vi "Plot area resize.vi"(8 "error in (no error)":errorcluster, 11 "Refs":T1) -> (0 "error out":errorcluster)   [LabVIEW 2021, in "RocketPlot.lvlib"]
uses:
  RocketPlot.lvlib
  TypeDefs/Plot UI references.ctl
  Classes/RocketPlotHandle/RocketPlotHandle.lvclass
  <userlib>/bjustice/TipStripOOPanel/Classes/TipPanelHandle/TipPanelHandle.lvclass
  TypeDefs/Plot top row.ctl
  TypeDefs/plotBG inputs.ctl
  <vilib>/Utility/miscctls.llb/LVBoundsTypeDef.ctl
  <vilib>/Utility/miscctls.llb/LVPositionTypeDef.ctl
  Plot scale refnum to LUT name.vi
  <vilib>/picture/picture.llb/Draw Rectangle.vi
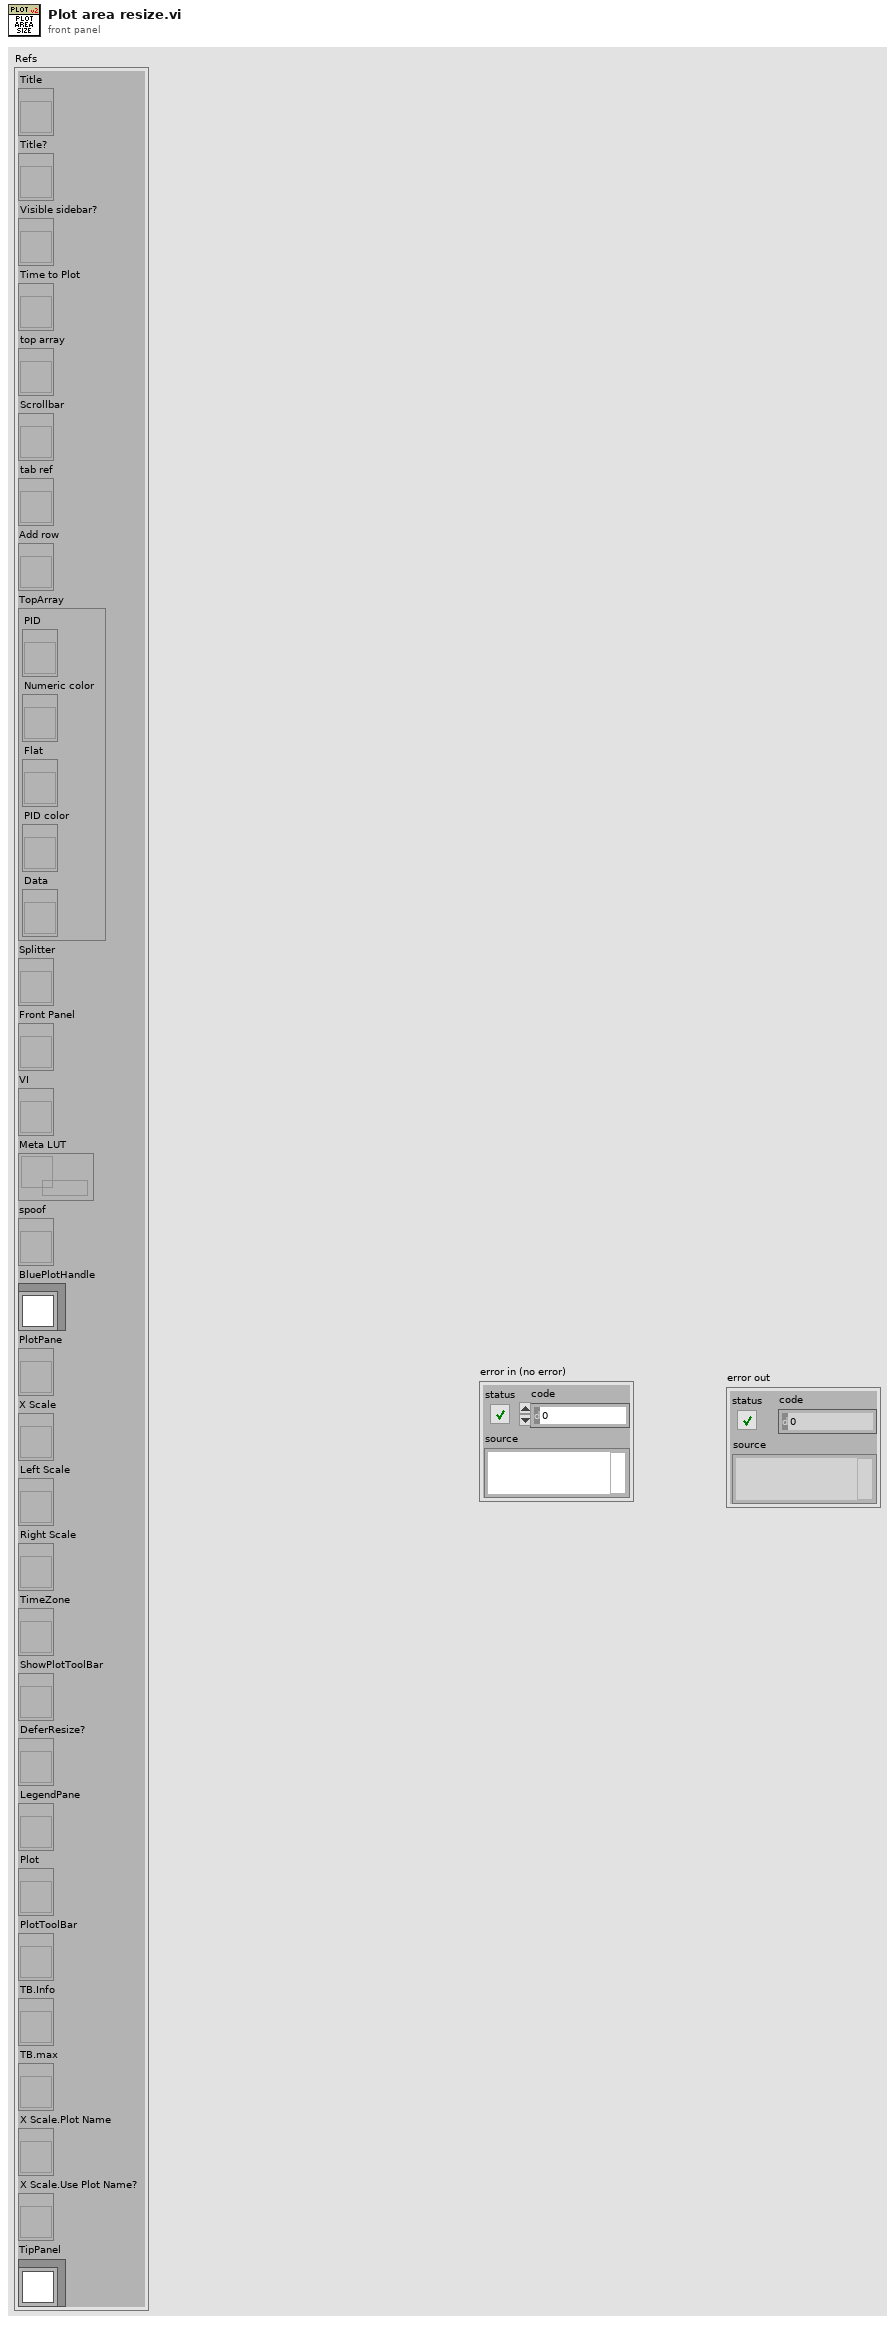
[diagram p1: front panel]
types:
  T1 = typedef "RocketPlot.lvlib/Plot UI references.ctl" = cluster{"Title":refnum<vi>, "Title?":refnum<vi>, "Visible sidebar?":refnum<vi>, "Time to Plot":refnum<vi>, "top array":refnum<vi>, "Scrollbar":refnum<vi>, "tab ref":refnum<vi>, "Add row":refnum<vi>, "TopArray":cluster{"PID":refnum<vi>, "Numeric color":refnum<vi>, "Flat":refnum<vi>, "PID color":refnum<vi>, "Data":refnum<vi>}, "Splitter":refnum<vi>, "Front Panel":refnum<vi>, "VI":refnum<vi>, "Meta LUT":refnum<data-value>, "spoof":refnum<vi>, "BluePlotHandle":refnum<class "RocketPlotHandle.lvclass">, "PlotPane":refnum<vi>, "X Scale":refnum<vi>, "Left Scale":refnum<vi>, "Right Scale":refnum<vi>, "TimeZone":refnum<vi>, "ShowPlotToolBar":refnum<vi>, "DeferResize?":refnum<vi>, "LegendPane":refnum<vi>, "Plot":refnum<vi>, "PlotToolBar":refnum<vi>, "TB.Info":refnum<vi>, "TB.max":refnum<vi>, "X Scale.Plot Name":refnum<vi>, "X Scale.Use Plot Name?":refnum<vi>, "TipPanel":refnum<class "TipPanelHandle.lvclass">}
  T2 = typedef "RocketPlot.lvlib/plotBG inputs.ctl" = cluster{"X.Scale Fit":u8, "Left.Scale Fit":u8, "Right.Scale Fit":u8}
  T3 = typedef "LVBoundsTypeDef.ctl" = cluster{"Width":u32, "Height":u32}
  T4 = typedef "LVPositionTypeDef.ctl" = cluster{"Left":i32, "Top":i32}
  T5 = typedef "RocketPlot.lvlib/Plot scale meta JSON.ctl" = cluster{"Type":T6, "Grid Colors:Major Color":u32, "Grid Colors:Minor Color":u32, "Style":u8, "Tick Colors:Tick Color":u32, "Tick Colors:Minor Tick Color":u32, "Format String":string, "State":T7, "AxisFocus":refnum<vi>}
  T6 = typedef "RocketPlot.lvlib/Plot axis.ctl" = enum16{"x axis", "left axis", "right axis"}
  T7 = typedef "RocketPlot.lvlib/Plot scale meta state.ctl" = cluster{"Visible":bool, "Focus":bool, "Multi-Y":bool}
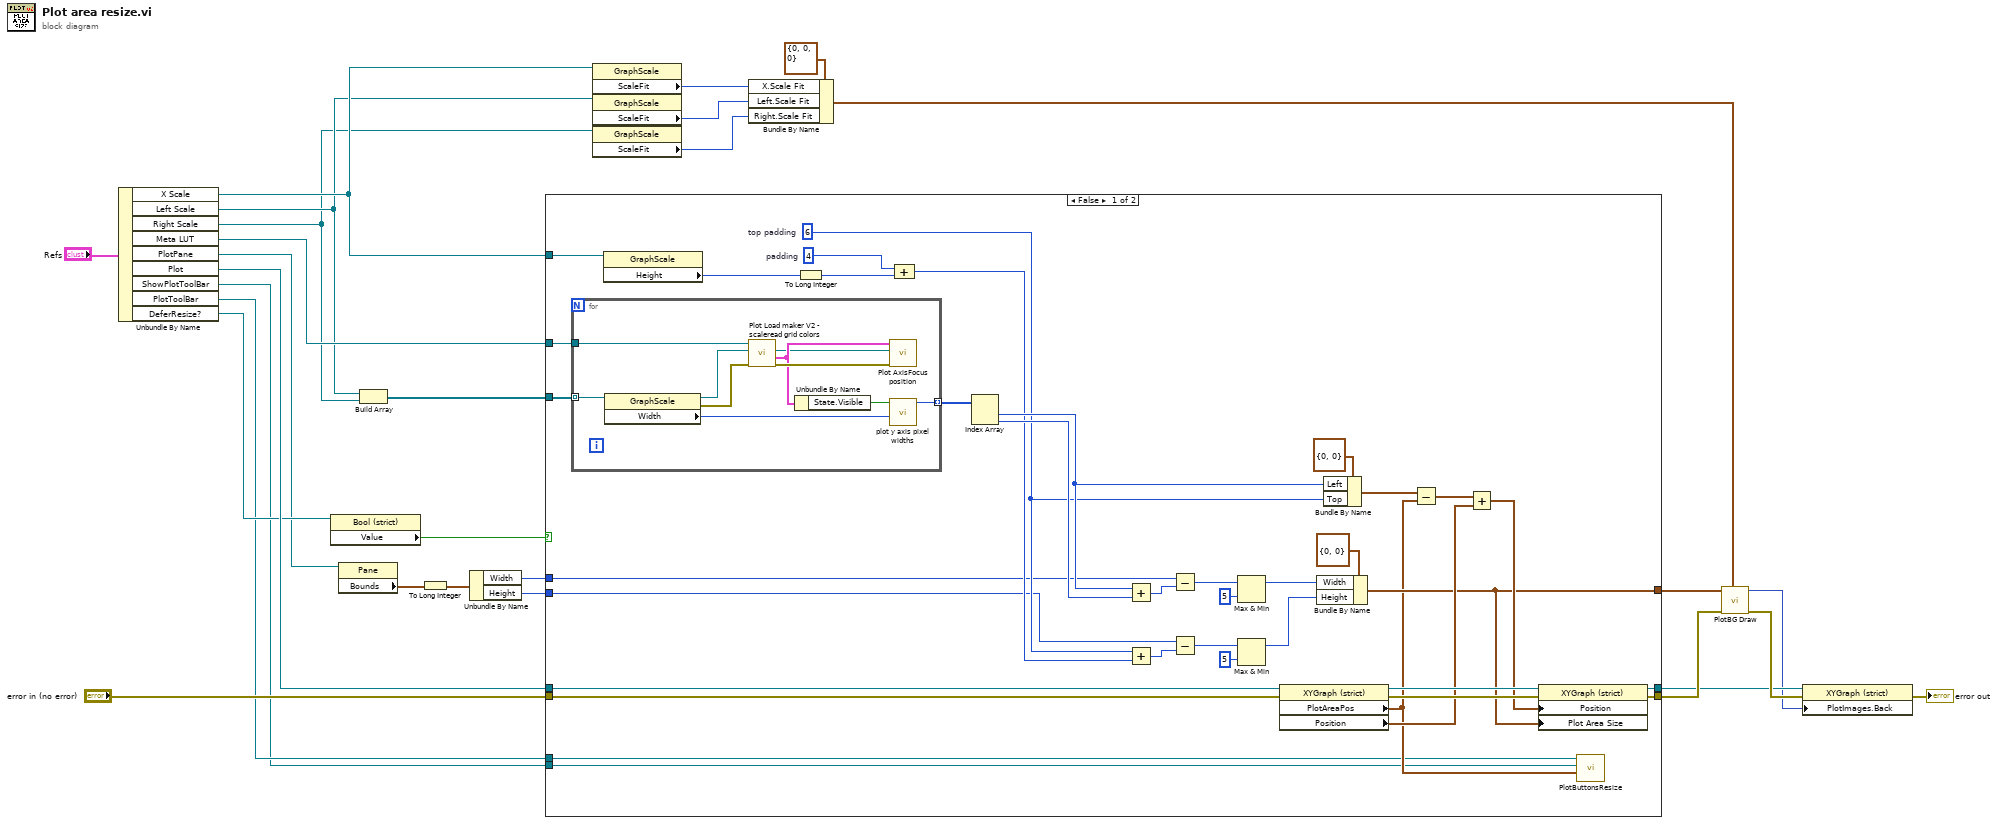
[diagram p0: block diagram]
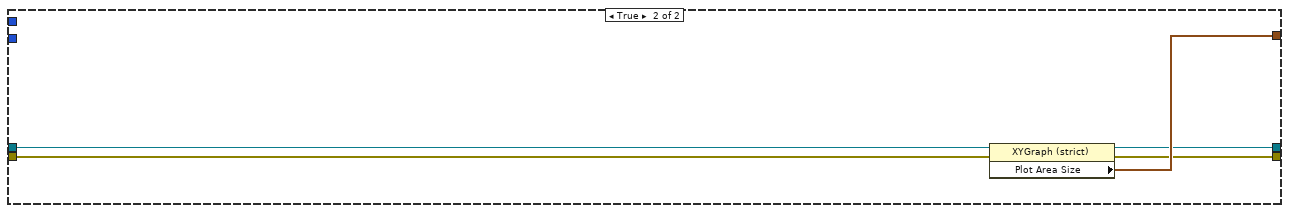
[diagram p2: hidden frame]
diagram:
  n1 = Unbundle By Name("Refs") -> ("X Scale"=w17:refnum<vi>, "Left Scale"=w16:refnum<vi>, "Right Scale"=w15:refnum<vi>, "Meta LUT"=w28:refnum<data-value>, "PlotPane"=w10:refnum<vi>, "Plot"=w23:refnum<vi>, "ShowPlotToolBar"=w1:refnum<vi>, "PlotToolBar"=w2:refnum<vi>, "DeferResize?"=w14:refnum<vi>)
  n2 = property class="Bool (strict)"(reference=w14) -> ("Value"=w13:bool)  [unwired: 1 in, 2 out]
  n3 = property class="Pane"(reference=w10) -> ("Bounds"=w11:T3)  [unwired: 1 in, 2 out]
  n4 = Build Array(w16, w15) -> (w24:refnum<vi>[])
  n5 = To Long Integer(number=w11) -> (32bit integer=w12:cluster{"Width":i32, "Height":i32})
  n6 = Unbundle By Name(w12) -> ("Width"=w9:i32, "Height"=w8:i32)
  n7 = case shown="False" w13 {
    tunnel: w28 -> [w65 _]
    tunnel: "error in (no error)" -> [w49 w78]
    tunnel: [w40 w77] -> w26
    tunnel: [w39 w79] -> w7
    tunnel: w24 -> [w37 _]
    tunnel: w23 -> [w36 w80]
    tunnel: w17 -> [w35 _]
    tunnel: w9 -> [w34 _]
    tunnel: w8 -> [w33 _]
    tunnel: [w32 w76] -> w5
    tunnel: w2 -> [w30 _]
    tunnel: w1 -> [w29 _]
    frame False {
      w51 = 4  # padding
      w54 = 6  # top padding
      n8 = for {
        tunnel: w65 -> [w75]
        tunnel: [w71] -> w64 mode=indexing
        tunnel: w37 -> [w69] mode=indexing
        n9 = property class="GraphScale"(reference=w69) -> (reference out=w74:refnum<vi>, error out=w73:errorcluster, "Width"=w70:u32)  [unwired: 1 in]
        n10 = call "Plot Load maker V2 - scaleread grid colors.vi"("error in (no error)"=w73, "Scale reference"=w74, "Meta LUT"=w75) -> ("error out"=w68:errorcluster, "Scale LUT meta"=w67:T5, "Scale reference"=w66:refnum<vi>)  [unwired: 5 in, 1 out]
        n11 = Unbundle By Name(w67) -> ("State.Visible"=w72:bool)
        n12 = call "Plot AxisFocus position.vi"("error in (no error)"=w68, "Scale reference"=w66, "Scale LUT meta"=w67) -> ()  [unwired: 8 in, 1 out]
        n13 = call "plot y axis pixel widths.vi"("Scale.Bounds:Area Width"=w70, "Axis.Visible"=w72) -> ("title width"=w71:i32)  [unwired: 9 in]
      }
      n14 = property class="GraphScale"(reference=w35) -> ("Height"=w41:u32)  [unwired: 1 in, 2 out]
      n15 = To Long Integer(number=w41) -> (32bit integer=w50:i32)
      n16 = Compound Arithmetic op=ADD(w51, w50) -> (w52:i32)
      n17 = Index Array(array=w64) -> (element #1=w57:i32, element #2=w56:i32)  [unwired: 2 in]
      n18 = Add(x=w57, y=w56) -> (x+y=w63:i32)
      n19 = Add(x=w54, y=w52) -> (x+y=w58:i32)
      n20 = Subtract(x=w34, y=w63) -> (x-y=w62:i32)
      n21 = Subtract(x=w33, y=w58) -> (x-y=w59:i32)
      n22 = Max & Min(x=w62, y=5) -> (max(x,y)=w55:i32)  [unwired: 1 out]
      n23 = Max & Min(x=w59, y=5) -> (max(x,y)=w53:i32)  [unwired: 1 out]
      n24 = property class="XYGraph (strict)"(reference=w36, error in=w49) -> (reference out=w48:refnum<vi>, error out=w47:errorcluster, "PlotAreaPos"=w31:T4, "Position"=w46:T4)
      n25 = Bundle By Name(cluster=T3 {"Width"=0, "Height"=0} ("Plot Area:Size"), "Width"=w55, "Height"=w53) -> (w39:T3)
      n26 = Bundle By Name(cluster=T4 {"Left"=0, "Top"=0} ("Position"), "Left"=w57, "Top"=w54) -> (w38:T4)
      n27 = Subtract(x=w38, y=w31) -> (x-y=w43:T4)
      n28 = Add(x=w43, y=w46) -> (x+y=w42:T4)
      n29 = property class="XYGraph (strict)"(reference=w48, error in=w47, "Position"=w42, "Plot Area Size"=w39) -> (reference out=w32:refnum<vi>, error out=w40:errorcluster)
      n30 = call "PlotButtonsResize.vi"("Plot Area:Position"=w31, "ShowPlotToolBar"=w29, "PlotToolBar"=w30) -> ()  [unwired: 8 in, 1 out]
    }
    frame True {
      n31 = property class="XYGraph (strict)"(reference=w80, error in=w78) -> (reference out=w76:refnum<vi>, error out=w77:errorcluster, "Plot Area Size"=w79:T3)
    }
  }
  n32 = property class="GraphScale"(reference=w17) -> ("ScaleFit"=w21:u8)  [unwired: 1 in, 2 out]
  n33 = property class="GraphScale"(reference=w16) -> ("ScaleFit"=w20:u8)  [unwired: 1 in, 2 out]
  n34 = property class="GraphScale"(reference=w15) -> ("ScaleFit"=w19:u8)  [unwired: 1 in, 2 out]
  n35 = Bundle By Name(cluster=T2 {"X.Scale Fit"=0, "Left.Scale Fit"=0, "Right.Scale Fit"=0} ("scale locked?"), "X.Scale Fit"=w21, "Left.Scale Fit"=w20, "Right.Scale Fit"=w19) -> (w18:T2)
  n36 = call "PlotBG Draw.vi"("scale locked?"=w18, "error in (no error)"=w26, "Draw Area Size"=w7) -> ("error out"=w6:errorcluster, "picture"=w3:picture)  [unwired: 7 in]
  n37 = property class="XYGraph (strict)"(reference=w5, error in=w6, "PlotImages.Back"=w3) -> (error out=→"error out":errorcluster)  [unwired: 1 out]
